vi "Square.vi"(11 "Side":dbl) -> (3 "Square Out":refnum<class "Square.lvclass">)   [LabVIEW 2018, in "Square.lvclass"]
uses:
  Square.lvclass
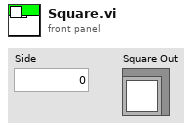
[diagram p1: front panel]
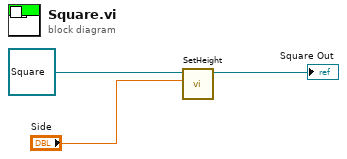
[diagram p0: block diagram]
diagram:
  n1 = call-dynamic "SetHeight.vi"("Height"="Side", "Square In"=refnum<class "Square.lvclass"> refnum ("Square in")) -> ("Square Out"=→"Square Out":refnum<class "Square.lvclass">)  [unwired: 9 in]
